vi "1dArrayTo2dArray.vi"(8 "error in (no error)":errorcluster, 10 "1D Array":dbl[](array[numeric]), 11 "MatOper in":refnum<class "MatOper.lvclass">) -> (0 "error out":errorcluster, 2 "2D Array":dbl[][](array[numeric]), 3 "MatOper out":refnum<class "MatOper.lvclass">)   [LabVIEW 2016, in "OfcFunc.lvlib" / "MatOper.lvclass"]
doc: "Reshape the 1D array (N elements) to 2D array (N x 1)."
uses:
  MatOper.lvclass
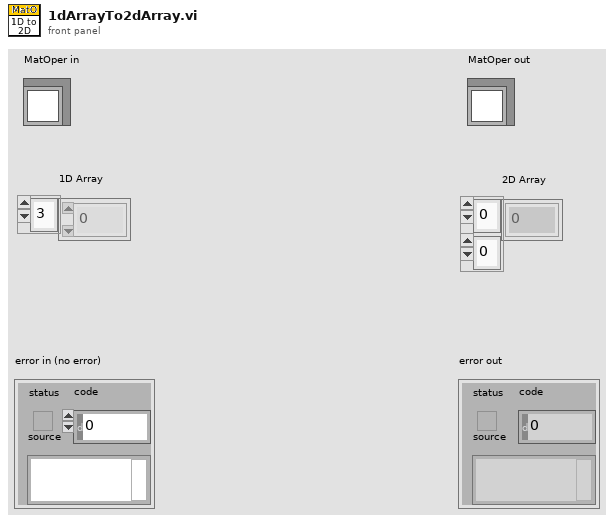
[diagram p1: front panel]
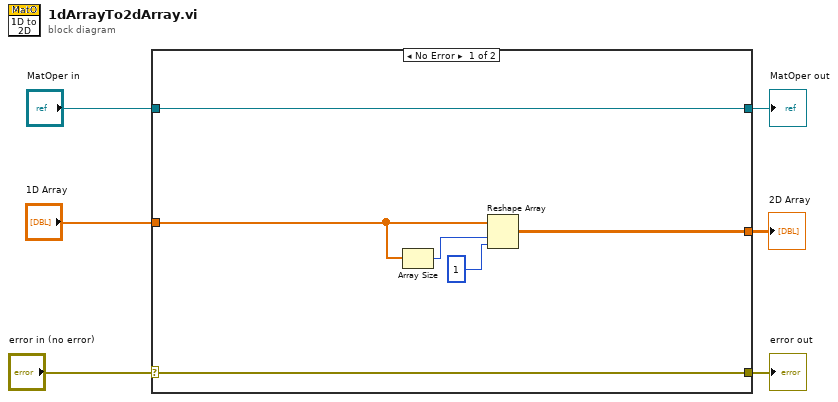
[diagram p0: block diagram]
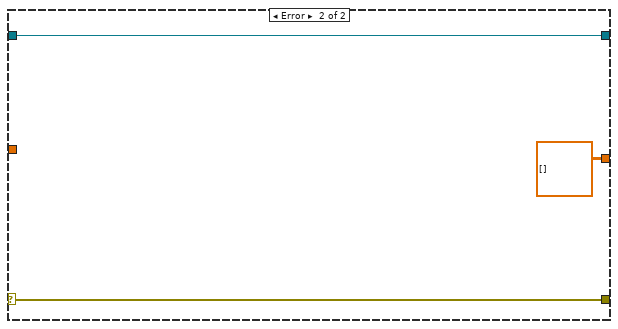
[diagram p2: hidden frame]
diagram:
  n1 = case shown="No Error" "error in (no error)" {
    selector: "error in (no error)" -> [w11 w15]
    tunnel: [w11 w15] -> w5
    tunnel: [w12 w14] -> w3
    tunnel: "MatOper in" -> [w12 w14]
    tunnel: "1D Array" -> [w8 _]
    tunnel: [w7 dbl[][] [] ("1D Array")] -> w1
    frame No Error {
      n2 = Array Size(array=w8) -> (size(s)=w9:i32)
      n3 = Reshape Array(w8, w9, 1 ("dimension size")) -> (w7:dbl[][])
    }
    frame Error {
    }
  }
  "error out" <- w5
  "MatOper out" <- w3
  "2D Array" <- w1
